vi "Set Position For Align Or Distribute.vi"(8 "Error In":errorcluster, 9 "Position":i32, 10 "Vertical? (F: Horizontal)":bool, 11 "Panel Object in":refnum<class "Panel Object.lvclass">) -> (0 "Error Out":errorcluster, 3 "Panel Object out":refnum<class "Panel Object.lvclass">)   [LabVIEW 2015, in "Panel Object.lvclass"]
uses:
  Panel Object.lvclass
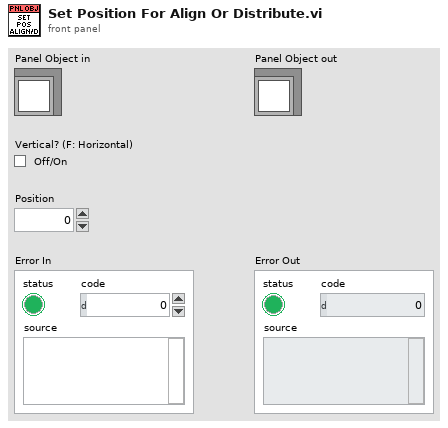
[diagram p1: front panel]
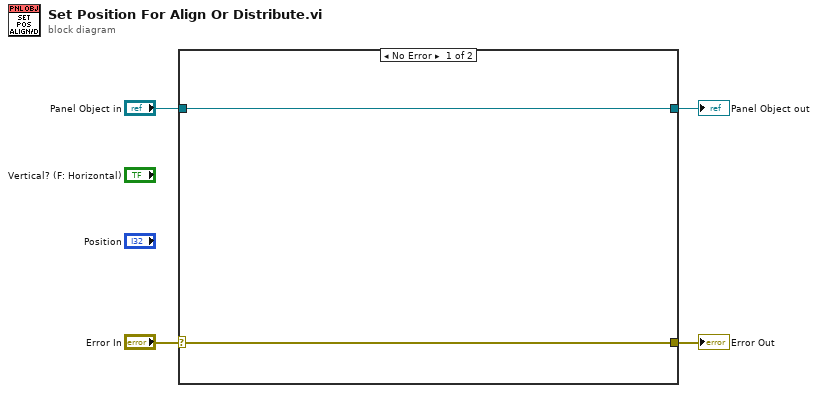
[diagram p0: block diagram]
diagram:
  n1 = case shown="No Error" "Error In" {
    selector: "Error In" -> [w5 w8]
    tunnel: [w5 w8] -> w1
    tunnel: [w6 w7] -> w3
    tunnel: "Panel Object in" -> [w6 w7]
    frame No Error {
    }
    frame Error {
    }
  }
  "Panel Object out" <- w3
  "Error Out" <- w1
